vi "Get Editor .NET.vi"(11 "Combo Box in":refnum<class "Combo Box.lvclass">) -> (2 "Editor Control .NET":refnum<k24>, 3 "Combo Box out":refnum<class "Combo Box.lvclass">)   [LabVIEW 2024, in "SourceGrid.lvlib" / "Combo Box.lvclass"]
uses:
  Combo Box.lvclass
  D:/git/Sourcegrid-LabVIEW/dll/SourceGrid.dll
  dll/SourceGrid.dll
  Combo Box.lvclass/Combo Box.ctl
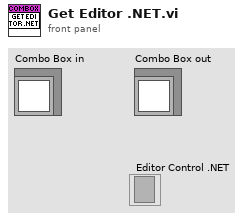
[diagram p1: front panel]
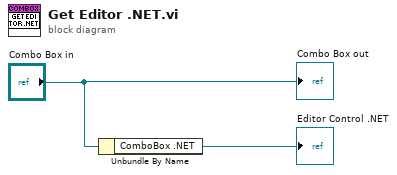
[diagram p0: block diagram]
diagram:
  n1 = Unbundle By Name("Combo Box in") -> ("ComboBox .NET"=→"Editor Control .NET":refnum<k24>)
  "Combo Box out" <- "Combo Box in"
